vi "Unflatten.vi"(8 "error in (no error)":errorcluster, 9 "timeout in":bool, 11 "CIFFifoCAN in":refnum<class "CIF_NIChn_FifoCAN.lvclass">) -> (0 "error out":errorcluster, 2 "Data":u8[](array[numeric]) format="%.0x", 3 "CIFFifoCAN out":refnum<class "CIF_NIChn_FifoCAN.lvclass">, 4 "Header":T1)   [LabVIEW 2021, in "CIF_NIChn_FifoCAN.lvclass"]
uses:
  CIF_NIChn_FifoCAN.lvclass
  CIF_NIChn_FifoCAN.lvclass/CIF_NIChn_FifoCAN.ctl
  ChannelCommon/CIFFIFO/CIFfifo.lvclass
  ChannelCommon/typedef/FIFO Header.ctl
  ChannelCommon/ChannelCommon.lvlib
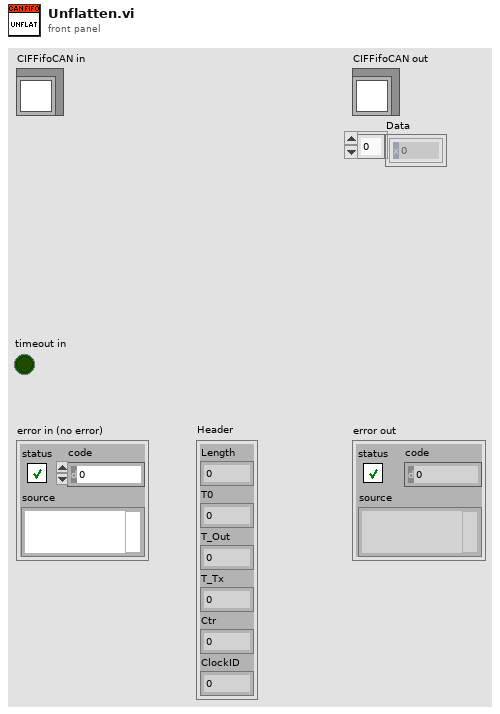
[diagram p1: front panel]
types:
  T1 = typedef "ChannelCommon.lvlib/FIFO Header.ctl" = cluster{"Length":u64, "T0":i64, "T_Out":i64, "T_Tx":i64, "Ctr":u64, "ClockID":u8}
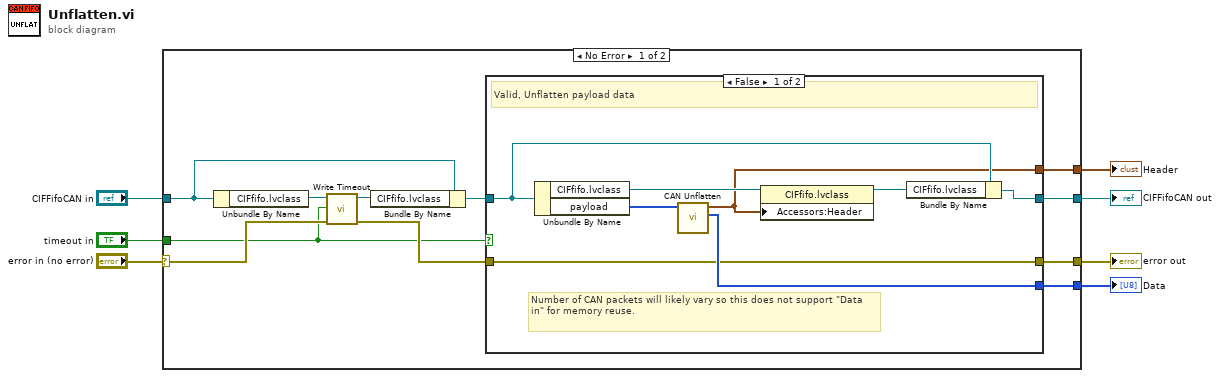
[diagram p0: block diagram]
diagram:
  n1 = case shown="No Error" "error in (no error)" {
    selector: "error in (no error)" -> [w17 w30]
    tunnel: [w11 w30] -> w6
    tunnel: [w12 w29] -> w4
    tunnel: "CIFFifoCAN in" -> [w18 w29]
    tunnel: "timeout in" -> [w10 _]
    tunnel: [w14 _] -> w1
    tunnel: [w13 _] -> w2
    frame No Error {
      n2 = Unbundle By Name(w18) -> ("CIFfifo.lvclass"=w9:refnum<class "CIFfifo.lvclass">)
      n3 = call "Write Timeout.vi"("error in (no error)"=w17, "Timeout"=w10, "CIFFIFO in"=w9) -> ("error out"=w16:errorcluster, "CIFFIFO out"=w8:refnum<class "CIFfifo.lvclass">)  [unwired: 7 in]
      n4 = Bundle By Name(cluster=w18, "CIFfifo.lvclass"=w8) -> (w15:refnum<class "CIF_NIChn_FifoCAN.lvclass">)
      n5 = case shown="False" w10 {
        tunnel: w16 -> [w19 w27]
        tunnel: w15 -> [w26 w28]
        tunnel: [w25 _] -> w14
        tunnel: [w20 _] -> w13
        tunnel: [w24 w28] -> w12
        tunnel: [w19 w27] -> w11
        frame False {
          # "Number of CAN packets will likely vary so this does not support \"Data in\" for memory reuse."
          # "Valid, Unflatten payload data"
          n6 = Unbundle By Name(w26) -> ("CIFfifo.lvclass"=w23:refnum<class "CIFfifo.lvclass">, "payload"=w21:u8[])
          n7 = call "CAN Unflatten.vi"("Flatten Data in"=w21) -> ("Data"=w25:u8[], "Header out"=w20:T1)  [unwired: 9 in]
          n8 = property class="CIFfifo.lvclass"(reference=w23, "Accessors:Header"=w20) -> (reference out=w22:refnum<class "CIFfifo.lvclass">)  [unwired: 1 in, 1 out]
          n9 = Bundle By Name(cluster=w26, "CIFfifo.lvclass"=w22) -> (w24:refnum<class "CIF_NIChn_FifoCAN.lvclass">)
        }
        frame True {
          # "Timeout"
        }
      }
    }
    frame Error {
    }
  }
  "error out" <- w6
  "CIFFifoCAN out" <- w4
  "Header" <- w2
  "Data" <- w1
